vi "Lake Shore 335 Configure Curve.vi"(0 "VISA resource name":refnum<visa-resource-name>="GPIB0::12::INSTR") -> ()   [LabVIEW 2017]
doc: "This VI was designed to demonstrate typical usage of sub VIs containing the more common 335 functions. The VI Initializes the instrument, allows the user to determine if heater output control parameters and setpoint values are sent, takes a single sensor reading, and then closes the instrument."
uses:
  <instrlib>/Lake Shore 335/Public/Data/Sensor Data (Single Reading).vi
  <vilib>/regexp/Match Regular Expression.xnode
  <instrlib>/Lake Shore 335/Lake Shore 335.lvlib
panel:
  in  "Display Mode (0:Input A)":u16(ring) items=["Input A", "Input A Max/Min", "Two Input, Loop A", "Input B", "Input B Max/Min", "Two Input, Loop B", "Custom", "Two Loop"]
  in  "Sensor":u16(ring) items=["NumSerie X64113", "NumSerie X71548"]
  in  "Configure Input Parameters":u16(ring) items=["Don't Configure", "Configure"]
  in  "Temperature Limit":u16=350
  in  "Enable \nCompensation":bool
  out "Curve":u16(ring)=21 items=["None"=0, "DT-470"=1, "DT-670"=2, "DT-500-D"=3, "DT-500-E1"=4, "PT-100"=6, "PT-1000"=7, "RX-102A-AA"=8, "RX-202A-AA"=9, "Type K"=12, "Type E"=13, "Type T"=14, "AuFe 0.03%"=15, "AuFe 0.07%"=16, "User 21"=21, "User 22"=22, "User 23"=23, "User 24"=24, "User 25"=25, "User 26"=26, "User 27"=27, "User 28"=28, "User 29"=29, "User 30"=30, "User 31"=31, "User 32"=32, "User 33"=33, "User 34"=34, "User 35"=35, "User 36"=36, "User 37"=37, "User 38"=38, "User 39"=39, "User 40"=40, "User 41"=41, "User 42"=42, "User 43"=43, "User 44"=44, "User 45"=45, "User 46"=46, "User 47"=47, "User 48"=48, "User 49"=49, "User 50"=50, "User 51"=51, "User 52"=52, "User 53"=53, "User 54"=54, "User 55"=55, "User 56"=56, "User 57"=57, "User 58"=58, "User 59"=59]
  in  "Preferred Units":u16(ring)=1 items=["Kelvin"=1, "Celsius"=2, "Sensor Units"=3]
  in  "Diode Current":u16(ring) items=["10 uA", "1 mA"]
  in  "Sensor Type and Range":u16(ring)=11 items=["Disabled", "Diode 2.5 V (Silicon)", "Diode 10 V (GaAlAs)", "PTC RTD Autorange", "PTC RTD 10 Ohm", "PTC RTD 30 Ohm", "PTC RTD 100 Ohm", "PTC RTD 300 Ohm", "PTC RTD 1 kOhm", "PTC RTD 3 kOhm", "PTC RTD 10 kOhm", "NTC RTD Autorange", "NTC RTD 10 Ohm", "NTC RTD 30 Ohm", "NTC RTD 100 Ohm", "NTC RTD 300 Ohm", "NTC RTD 1 kOhm", "NTC RTD 3 kOhm", "NTC RTD 10 kOhm", "NTC RTD 30 kOhm", "NTC RTD 100 kOhm", "Thermocouple"]
  in  "Input":u16(ring) items=["A", "B"]
  out "Input Name (\"\")":string="miSensor"
  in  "Polarity (0:Unipolar)":u16(ring) items=["Unipolar", "Bipolar"]
  in  "Output Type (0:Current)":u16(ring) items=["Current", "Voltage"]
  in  "Heater Output (1:1)":u16(ring)=1 items=["1"=1, "2"=2]
  in  "Heater Resistance (1:25 Ohm)":u16(ring)=2 items=["25 Ohm"=1, "50 Ohm"=2]
  in  "Max User Current (1.732)":dbl=1.732 format="%.3f"
  in  "Heater Out Display (1:Current)":u16(ring)=1 items=["Current"=1, "Power"=2]
  in  "Max Current (0:User Specified)":u16(ring)=2 items=["User Specified", "0.707 A", "1.0 A", "1.141 A", "1.732 A"]
  in  "Mode (0:Off)":u16(ring)=1 items=["Off", "Closed Loop PID", "Zone", "Open Loop", "Monitor Out", "Warmup Supply"]
  in  "Power Up Enable (F: Off)":bool
  in  "Input (0:None)":u16(ring)=1 items=["None", "A", "B"]
  in  "Input":u16(ring) items=["A", "B"]
  in  "Data Source":u16(ring) items=["Kelvin", "Celsius", "Sensor Units"]
  out "Sensor Data":dbl format="%.4f"
  in  "Configure Setpoint":u16(ring) items=["Don't Configure", "Configure"]
  in  "Setpoint":dbl format="%.4f"
  in  "Manual Output (0.00 %)":dbl format="%.2f"
  in  "Range (0:Off)":u16(ring) items=["Off", "Low (On)", "Medium", "High"]
  in  "Rate (D) (0.0 %)":dbl format="%.1f"
  in  "Reset (I) (20.0)":dbl=20.0 format="%.1f"
  in  "Gain (P) (50.0)":dbl=50.0 format="%.1f"
  in  "Serial Configuration":T1={"Baud Rate"=57600, "Parity"=1, "Data Bits"=7, "Stop Bits"=10, "Flow Control"=0} {"Flow Control" items=["None", "XON/XOFF", "RTS/CTS", "XON/XOFF & RTS/CTS", "DTR/DSR", "XON/XOFF & DTR/DSR"]; "Stop Bits" items=["1.0"=10, "1.5"=15, "2.0"=20]; "Data Bits" items=["7"=7, "8"=8]; "Parity" items=["None", "Odd", "Even", "Mark", "Space"]; "Baud Rate" items=["300"=300, "600"=600, "1200"=1200, "2400"=2400, "4800"=4800, "9600"=9600, "19200"=19200, "38400"=38400, "57600"=57600]}
  in  "Configure Control Parameters":u16(ring) items=["Don't Configure", "Configure"]
  # "Configurar curva para sensor A.\nSeleccionar sensor y ejecutar programa"
  # "(c) 2011 Lake Shore Cryotronics Inc.  ALL RIGHTS RESERVED."
  # "(c) 2020 SIE.SAI MODIFICADO.  ALL RIGHTS RESERVED."
  # "Input Parameters"
  # "Output Setpoint"
  # "Sensor Data"
  # "Output Control Parameters"
  # "Settings for Either Heater Output"
  # "Settings for Heater Output 2 Only"
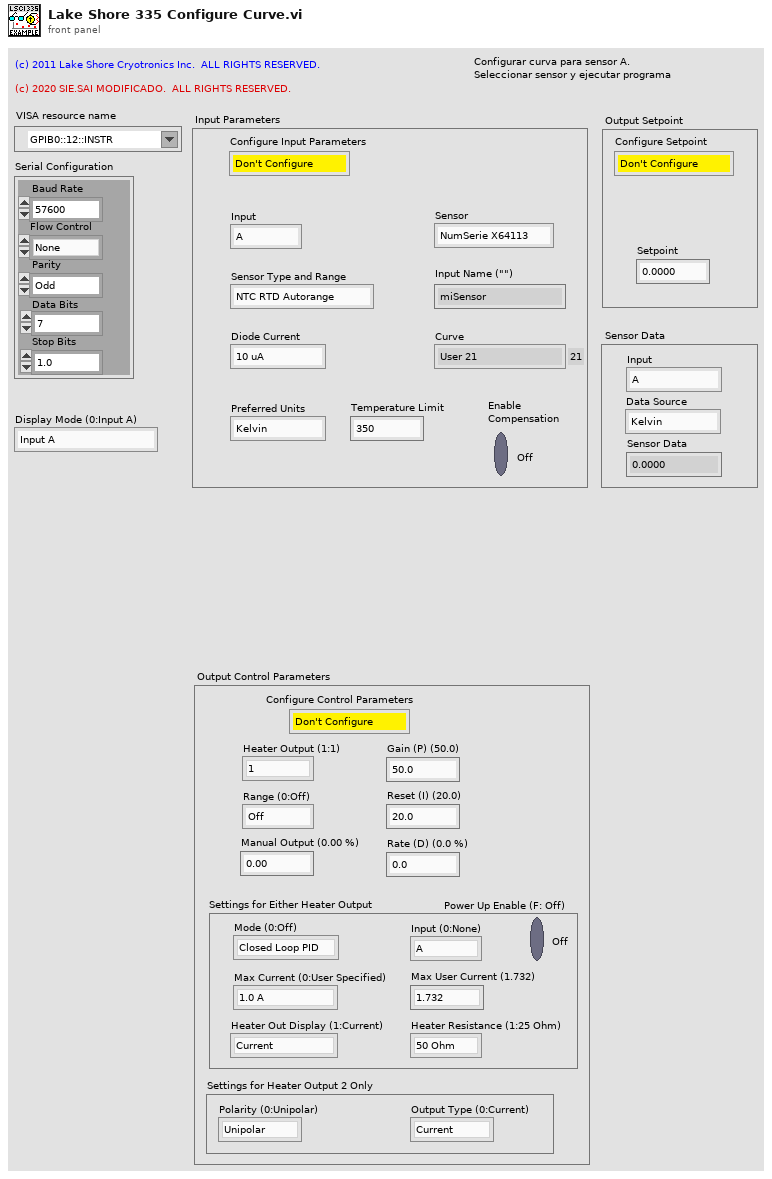
[diagram p1: front panel]
types:
  T1 = cluster{"Baud Rate":u32, "Parity":u16, "Data Bits":u16, "Stop Bits":u16, "Flow Control":u16}
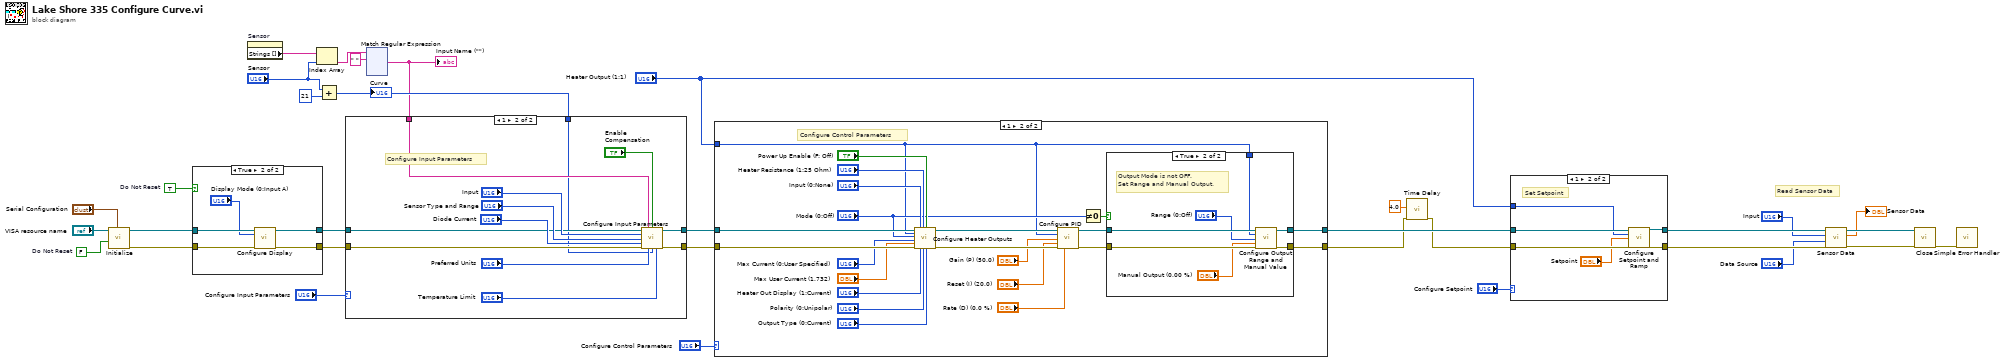
[diagram p0: block diagram]
diagram:
  w4 = TRUE  # Do Not Reset
  w29 = FALSE  # Do Not Reset
  # "Read Sensor Data"
  n1 = call <instrlib>:"Initialize.vi"("Serial Configuration"="Serial Configuration", "Reset (True)"=w29, "VISA resource name"="VISA resource name") -> ("error out"=w8:errorcluster, "VISA resource name out"=w6:refnum<visa-resource-name>)  [unwired: 7 in]
  n2 = case shown="True" w4 {
    tunnel: w8 -> [w34 w40]
    tunnel: [w34 w39] -> w7
    tunnel: w6 -> [w35 w38]
    tunnel: [w35 w37] -> w5
    frame False {
    }
    frame True {
      n3 = call <instrlib>:"Configure Display.vi"("VISA resource name"=w38, "Display Mode (0:Input A)"="Display Mode (0:Input A)", "error in (no error)"=w40) -> ("VISA resource name out"=w37:refnum<visa-resource-name>, "error out"=w39:errorcluster)  [unwired: 11 in]
    }
  }
  n4 = property on="Sensor" class="Ring (strict)"() -> ("Strings []"=w15:string[])  [unwired: 2 in, 2 out]
  n5 = Index Array(array=w15, index="Sensor") -> (element=w10:string)
  n6 = Add(x="Sensor", y=u16 21) -> (x+y=w12:u16)
  "Curve" <- w12
  n7 = xnode "Match Regular Expression"("input string"=w10, "regular expression"=" ") -> ("after match"=w9:string)  [unwired: 4 in, 4 out]
  "Input Name (\"\")" <- w9
  n8 = case shown="1" "Configure Input Parameters" {
    tunnel: w5 -> [w42 w48]
    tunnel: w7 -> [w41 w47]
    tunnel: [w41 w46] -> w17
    tunnel: [w42 w45] -> w16
    tunnel: w9 -> [_ w44]
    tunnel: w12 -> [_ w43]
    frame 0, Default {
      # "Do Not Configure Input Parameters"
    }
    frame 1 {
      # "Configure Input Parameters"
      n9 = call <instrlib>:"Configure Input Parameters.vi"("VISA resource name"=w48, "Input Name (\"\")"=w44, "Enable \nCompensation (F: Off)"="Enable \nCompensation", "Input (0:A)"="Input", "Sensor Type and Range (0:Disabled)"="Sensor Type and Range", "Diode Current (0:10 uA)"="Diode Current", "error in (no error)"=w47, "Preferred Units (1:Kelvin)"="Preferred Units", "Curve (0:None)"=w43, "Temperature Limit (0)"="Temperature Limit") -> ("VISA resource name out"=w45:refnum<visa-resource-name>, "error out"=w46:errorcluster)  [unwired: 4 in]
    }
  }
  n10 = case shown="1" "Configure Control Parameters" {
    tunnel: "Heater Output (1:1)" -> [_ w57]
    tunnel: w16 -> [w56 w72]
    tunnel: w17 -> [w55 w71]
    tunnel: [w55 w76] -> w2
    tunnel: [w56 w75] -> w30
    frame 0, Default {
      # "Do Not Configure Control Parameters"
    }
    frame 1 {
      # "Configure Control Parameters"
      n11 = call <instrlib>:"Configure Heater Outputs.vi"("VISA resource name"=w72, "Heater Output (1:1)"=w57, "Mode (0:Off)"="Mode (0:Off)", "Max Current (0:User Specified)"="Max Current (0:User Specified)", "Max User Current (1.732)"="Max User Current (1.732)", "error in (no error)"=w71, "Input (0:None)"="Input (0:None)", "Heater Out Display (1:Current)"="Heater Out Display (1:Current)", "Heater Resistance (1:25 Ohm)"="Heater Resistance (1:25 Ohm)", "Polarity (0:Unipolar)"="Polarity (0:Unipolar)", "Power Up Enable (F: Off)"="Power Up Enable (F: Off)", "Output Type (0:Current)"="Output Type (0:Current)") -> ("VISA resource name out"=w74:refnum<visa-resource-name>, "error out"=w73:errorcluster)  [unwired: 6 in]
      n12 = call <instrlib>:"Configure PID.vi"("VISA resource name"=w74, "Output's Control Loop (1:1)"=w57, "Gain (P) (50.0)"="Gain (P) (50.0)", "Reset (I) (20.0)"="Reset (I) (20.0)", "error in (no error)"=w73, "Rate (D) (0.0 %)"="Rate (D) (0.0 %)") -> ("VISA resource name out"=w78:refnum<visa-resource-name>, "error out"=w77:errorcluster)  [unwired: 8 in]
      n13 = Not Equal To 0?(x="Mode (0:Off)") -> (x != 0?=w67:bool)
      n14 = case shown="True" w67 {
        tunnel: w78 -> [w80 w87]
        tunnel: w77 -> [w79 w86]
        tunnel: [w79 w85] -> w76
        tunnel: [w80 w84] -> w75
        tunnel: w57 -> [_ w83]
        frame False {
          # "Output Mode is OFF.  Do not\nset Range and Manual Output (prevents \nExecution Error)."
        }
        frame True {
          # "Output Mode is not OFF.\nSet Range and Manual Output."
          n15 = call <instrlib>:"Configure Output Range and Manual Value.vi"("VISA resource name"=w87, "Heater Output (1:1)"=w83, "Range (0:Off)"="Range (0:Off)", "Manual Output (0.00 %)"="Manual Output (0.00 %)", "error in (no error)"=w86) -> ("VISA resource name out"=w84:refnum<visa-resource-name>, "error out"=w85:errorcluster)  [unwired: 9 in]
        }
      }
    }
  }
  n16 = call "Time Delay"("error in (no error)"=w2, "Delay Time (s)"=4.0) -> ("error out"=w3:errorcluster)  [unwired: 9 in]
  n17 = case shown="1" "Configure Setpoint" {
    tunnel: "Heater Output (1:1)" -> [_ w93]
    tunnel: w30 -> [w89 w94]
    tunnel: w3 -> [w88 w95]
    tunnel: [w88 w91] -> w26
    tunnel: [w89 w92] -> w27
    frame 0, Default {
      # "Do Not Set Setpoint"
    }
    frame 1 {
      # "Set Setpoint"
      n18 = call <instrlib>:"Configure Setpoint and Ramp.vi"("VISA resource name"=w94, "Output's Control Loop (1:1)"=w93, "Setpoint (0.0000)"="Setpoint", "error in (no error)"=w95) -> ("VISA resource name out"=w92:refnum<visa-resource-name>, "error out"=w91:errorcluster)  [unwired: 10 in]
    }
  }
  n19 = call-poly <instrlib>:"Sensor Data.vi"("error in (no error)"=w26, "Data Source (0:Kelvin)"="Data Source", "Input (0:A)"="Input", "VISA resource name"=w27) -> ("error out"=w24:errorcluster, "Sensor Data"=→"Sensor Data":dbl, "VISA resource name out"=w25:refnum<visa-resource-name>)  [unwired: 5 in]
  n20 = call <instrlib>:"Close.vi"("error in (no error)"=w24, "VISA resource name"=w25) -> ("error out"=w31:errorcluster)  [unwired: 9 in]
  n21 = call <vilib>:"Simple Error Handler.vi"("error in (no error)"=w31) -> ()  [unwired: 4 in, 5 out]
